vi "exp2_函数发生器.vi"() -> ()   [LabVIEW 2021]
uses:
  <vilib>/Analysis/NI_AALBase.lvlib
panel:
  out "波形数据":waveform(dbl)
  in  "停止":bool
  in  "波形选择":enum16{"正弦波", "三角波", "方波", "锯齿波"}(ring)
  in  "延时选择":i16
  in  "占空比（%）":i8
  in  "初始相位":sgl
  in  "直流偏移":sgl
  in  "采样频率（Hz）":sgl
  in  "频率（Hz）":dbl
  in  "幅度（V）":sgl
  in  "采样点数":i32
  out "监视器":waveform(dbl)(graph)
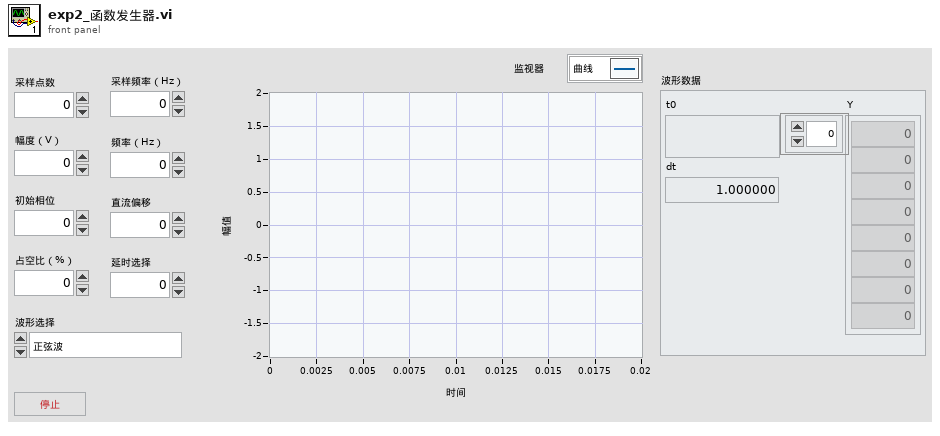
[diagram p1: front panel]
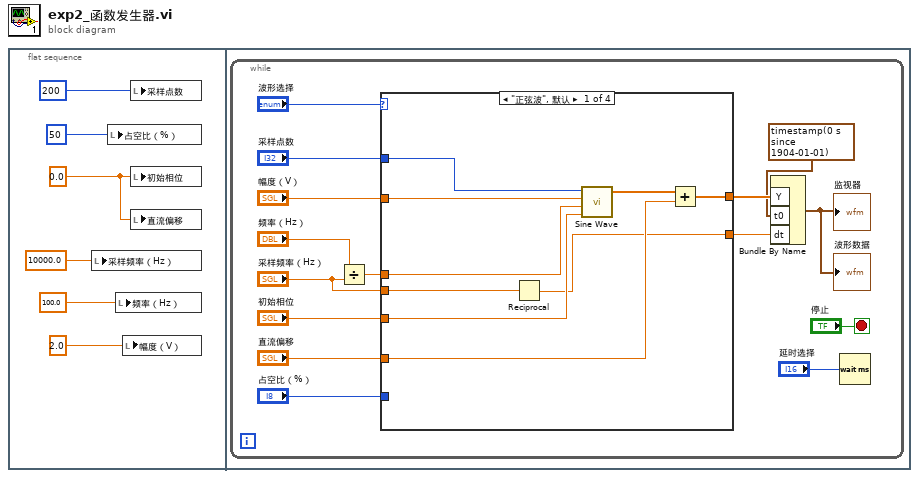
[diagram p0: block diagram]
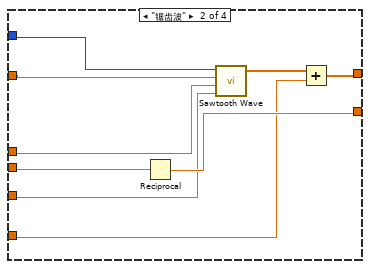
[diagram p2: hidden frame]
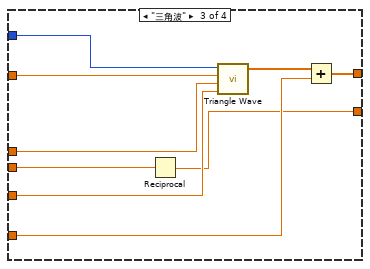
[diagram p3: hidden frame]
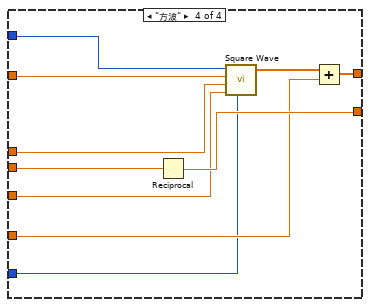
[diagram p4: hidden frame]
diagram:
  n1 = flat-sequence {
    frame #0 {
      w6 = 0.0
      n2 = local write "采样频率（Hz）"(10000.0) -> ()
      n3 = local write "占空比（%）"(50) -> ()
      n4 = local write "频率（Hz）"(100.0) -> ()
      n5 = local write "幅度（V）"(2.0) -> ()
      n6 = local write "采样点数"(200) -> ()
      n7 = local write "初始相位"(w6) -> ()
      n8 = local write "直流偏移"(w6) -> ()
    }
    frame #1 {
      n9 = while {
        stop <- "停止" stop-if-true
        n10 = Divide(x="频率（Hz）", y="采样频率（Hz）") -> (x/y=w9:dbl)
        n11 = case shown="\"正弦波\", 默认" "波形选择" {
          tunnel: "初始相位" -> [w30 w35 w43 w54]
          tunnel: "幅度（V）" -> [w29 w31 w46 w50]
          tunnel: "采样点数" -> [w28 w32 w47 w51]
          tunnel: "采样频率（Hz）" -> [w27 w34 w44 w53]
          tunnel: "直流偏移" -> [w26 w36 w42 w55]
          tunnel: [w24 w38 w40 w56] -> w12
          tunnel: [w23 w37 w41 w57] -> w10
          tunnel: w9 -> [w22 w33 w45 w52]
          tunnel: "占空比（%）" -> [_ _ _ w49]
          frame "正弦波", Default {
            n12 = Reciprocal(x=w27) -> (1/x=w23:sgl)
            n13 = call <vilib>:"Sine Wave.vi"("samples"=w28, "amplitude"=w29, "frequency"=w22, "phase in"=w30) -> ("sine wave"=w25:dbl[])  [unwired: 1 in, 2 out]
            n14 = Add(x=w25, y=w26) -> (x+y=w24:dbl[])
          }
          frame "锯齿波" {
            n15 = Reciprocal(x=w34) -> (1/x=w37:sgl)
            n16 = call <vilib>:"Sawtooth Wave.vi"("samples"=w32, "amplitude"=w31, "frequency"=w33, "phase in"=w35) -> ("sawtooth wave"=w39:dbl[])  [unwired: 1 in, 2 out]
            n17 = Add(x=w39, y=w36) -> (x+y=w38:dbl[])
          }
          frame "三角波" {
            n18 = Reciprocal(x=w44) -> (1/x=w41:sgl)
            n19 = call <vilib>:"Triangle Wave.vi"("samples"=w47, "amplitude"=w46, "frequency"=w45, "phase in"=w43) -> ("triangle wave"=w48:dbl[])  [unwired: 1 in, 2 out]
            n20 = Add(x=w48, y=w42) -> (x+y=w40:dbl[])
          }
          frame "方波" {
            n21 = Reciprocal(x=w53) -> (1/x=w57:sgl)
            n22 = call <vilib>:"Square Wave.vi"("samples"=w51, "amplitude"=w50, "frequency"=w52, "duty cycle (%)"=w49, "phase in"=w54) -> ("square wave"=w58:dbl[])  [unwired: 1 in, 2 out]
            n23 = Add(x=w58, y=w55) -> (x+y=w56:dbl[])
          }
        }
        n24 = Bundle By Name("Y"=w12, "t0"=timestamp(0 s since 1904-01-01), "dt"=w10) -> (→"监视器" →"波形数据":waveform(dbl))  [unwired: 1 in]
        n25 = Wait (ms)(milliseconds to wait="延时选择") -> ()  [unwired: 1 out]
      }
    }
  }
